vi "SHA-1.vi"(10 "data":u8[](array[numeric]) format="%02x") -> (2 "SHA-1 hash":u8[](array[numeric]) format="%02x")   [LabVIEW 2013, in "SHA-1.lvlib"]
uses:
  SHA-1.lvlib
  SHA-1.lvclass
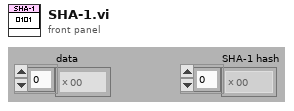
[diagram p1: front panel]
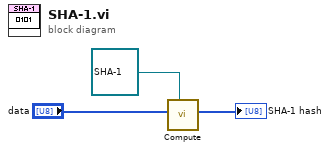
[diagram p0: block diagram]
diagram:
  n1 = call-dynamic "Compute.vi"("SHA-1"=refnum<class "SHA-1.lvclass"> refnum, "data"="data") -> ("hash"=→"SHA-1 hash":u8[])  [unwired: 9 in]
